vi "ST5 Wait Stop.vi"(8 "error in":errorcluster, 9 "Move Ref":refnum<vi>, 10 "Delay(s)":i32=40, 11 "Port COM":refnum<visa-resource-name>) -> (0 "error out":errorcluster, 3 "Port Out":refnum<visa-resource-name>)   [LabVIEW 2010]
uses:
  <userlib>/GenProg/ReadbyWeakRefBool.vi
panel:
  in  "Stop":bool
  out "read buffer":string
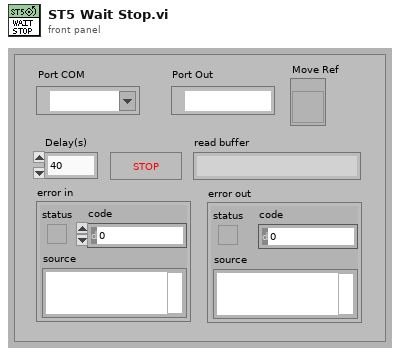
[diagram p1: front panel]
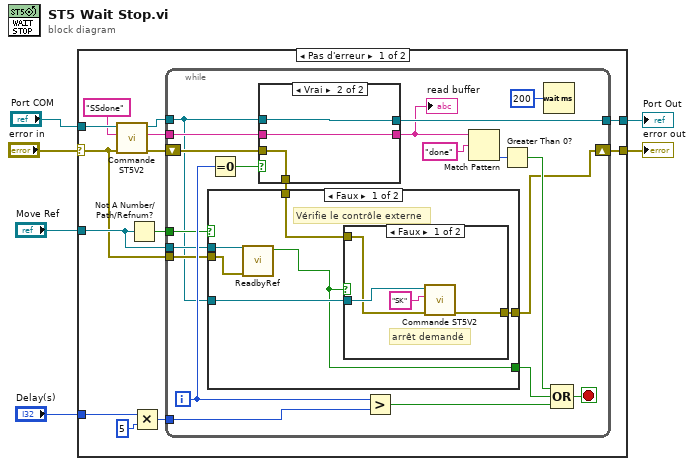
[diagram p0: block diagram]
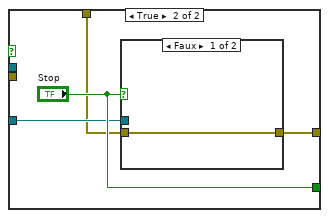
[diagram p3: hidden frame]
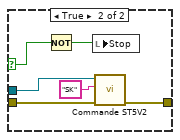
[diagram p4: hidden frame]
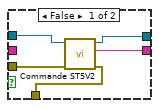
[diagram p5: hidden frame]
diagram:
  n1 = case shown="Pas d'erreur" "error in" {
    selector: "error in" -> [w7 w71]
    tunnel: [w19 w71] -> w6
    tunnel: "Port COM" -> [w17 w70]
    tunnel: [w13 w70] -> w4
    tunnel: "Delay(s)" -> [w12 _]
    tunnel: "Move Ref" -> [w8 _]
    frame No Error {
      n2 = call <userlib>:"Commande ST5V2.vi"("error in (no error)"=w7, "Commande"="SSdone" ("write buffer"), "Port COM"=w17) -> ("error out"=w18:errorcluster, "Réponse"=w14:string, "Port Out"=w16:refnum<visa-resource-name>)  [unwired: 2 in]
      n3 = Not A Number/Path/Refnum?(number/path/refnum=w8) -> (NaN/Path/Refnum?=w9:bool)
      n4 = Multiply(x=w12, y=5) -> (x*y=w10:i32)
      n5 = while {
        tunnel: w16 -> [w22]
        shift-right: [w20] -> w19
        shift-left: w18 -> [w35]
        tunnel: w14 -> [w34]
        tunnel: [w32] -> w13
        tunnel: w10 -> [w31]
        tunnel: w9 -> [w29]
        tunnel: w8 -> [w30]
        tunnel: w7 -> [w25]
        i -> [w36]
        stop <- w26 stop-if-true
        n6 = Equal To 0?(x=w36) -> (x = 0?=w33:bool)
        n7 = case shown="Vrai" w33 {
          tunnel: w35 -> [w66 w69]
          tunnel: w22 -> [w65 w67]
          tunnel: w34 -> [_ w68]
          tunnel: [w62 w69] -> w21
          tunnel: [w64 w68] -> w24
          tunnel: [w63 w67] -> w32
          frame False {
            n8 = call <userlib>:"Commande ST5V2.vi"("error in (no error)"=w66, "Port COM"=w65) -> ("error out"=w62:errorcluster, "Réponse"=w64:string, "Port Out"=w63:refnum<visa-resource-name>)  [unwired: 3 in]
          }
          frame True {
          }
        }
        "read buffer" <- w24
        n9 = case shown="Faux" w29 {
          tunnel: w30 -> [w42 _]
          tunnel: [w41 "Stop"] -> w28
          tunnel: w25 -> [w40 _]
          tunnel: w22 -> [w45 w53]
          tunnel: w21 -> [w43 w52]
          tunnel: [w44 w51] -> w20
          frame False {
            # "Vérifie le contrôle externe"
            n10 = call-poly <userlib>:"ReadbyRef.vi"("error in"=w40, "Control Ref"=w42) -> ("Valeur"=w41:bool)  [unwired: 8 in, 1 out]
            n11 = case shown="Faux" w41 {
              tunnel: w45 -> [w48 _]
              tunnel: [w47 w50] -> w44
              tunnel: w43 -> [w46 w50]
              frame False {
                # "arrêt demandé"
                n12 = call <userlib>:"Commande ST5V2.vi"("error in (no error)"=w46, "Commande"="SK", "Port COM"=w48) -> ("error out"=w47:errorcluster)  [unwired: 2 in, 2 out]
              }
              frame True {
              }
            }
          }
          frame True {
            n13 = case shown="Faux" "Stop" {
              selector: "Stop" -> [_ w60]
              tunnel: w53 -> [_ w58]
              tunnel: w52 -> [w55 w57]
              tunnel: [w55 w56] -> w51
              frame False {
              }
              frame True {
                n14 = Not(x=w60) -> (.not. x?=w61:bool)
                n15 = local write "Stop"(w61) -> ()
                n16 = call <userlib>:"Commande ST5V2.vi"("error in (no error)"=w57, "Commande"="SK", "Port COM"=w58) -> ("error out"=w56:errorcluster)  [unwired: 2 in, 2 out]
              }
            }
          }
        }
        n17 = Greater?(x=w36, y=w31) -> (0:w23:bool)
        n18 = Match Pattern(string=w24, regular expression="done") -> (offset past match=w37:i32)  [unwired: 1 in, 3 out]
        n19 = Greater Than 0?(x=w37) -> (x > 0?=w27:bool)
        n20 = Wait (ms)(milliseconds to wait=u32 200) -> ()  [unwired: 1 out]
        n21 = Compound Arithmetic op=OR(w27, w28, w23) -> (w26:bool)
      }
    }
    frame Error {
    }
  }
  "error out" <- w6
  "Port Out" <- w4
